vi "Calibrate Input.vi"(0 "VISA resource name":refnum<visa-resource-name>, 1 "Unit Address (1)":i16=1, 5 "Input (1)":i16=1, 7 "Calibration (0: 0.00 mV Thermocouple)":u16(ring) items=["0.00 mV Thermocouple", "50.00 mV Thermocouple", "32°F Type J", "Ground", "Lead", "15.0 Ohms", "240.0 Ohms", "380.0 Ohms", "6080.0 Ohms", "0.000 V", "10.000 V", "4.000 mA", "20.000 mA"], 11 "error in (no error)":errorcluster {"code" format="%.0x"}) -> (4 "VISA resource name out":refnum<visa-resource-name>, 15 "error out":errorcluster {"code" format="%.0x"})   [LabVIEW 2010]
doc: "This VI sets calibration input."
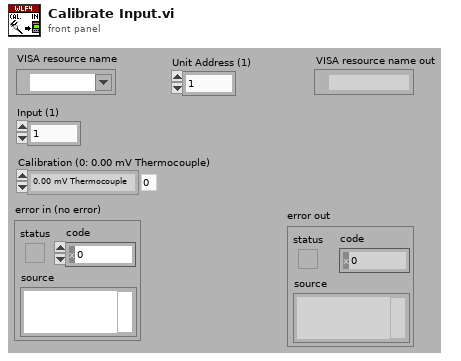
[diagram p1: front panel]
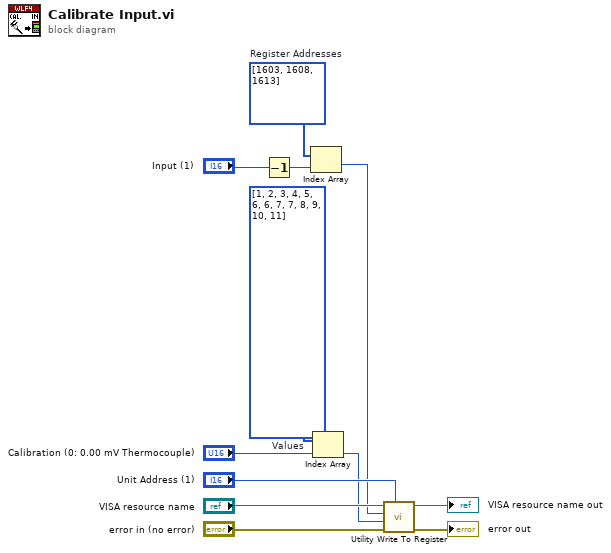
[diagram p0: block diagram]
diagram:
  w2 = i32[] [1, 2, 3, 4, 5, 6, 6, 7, 7, 8, 9, 10, 11]  # Values
  w7 = i32[] [1603, 1608, 1613]  # Register Addresses
  n1 = Decrement(x="Input (1)") -> (x-1=w5:i16)
  n2 = Index Array(array=w7, index=w5) -> (element=w4:i32)
  n3 = Index Array(array=w2, index="Calibration (0: 0.00 mV Thermocouple)") -> (element=w3:i32)
  n4 = call "Utility Write To Register.vi"("Unit Address (1)"="Unit Address (1)", "error in (no error)"="error in (no error)", "Data (0)"=w3, "Register Address (0)"=w4, "VISA resource name"="VISA resource name") -> ("error out"=→"error out":errorcluster, "VISA resource name out"=→"VISA resource name out":refnum<visa-resource-name>)  [unwired: 5 in]
